vi "BLAS1 Utility(DBL).vi"(0 "x":dbl[](array[numeric]), 1 "y":dbl[](array[numeric]), 2 "xInc":i32, 3 "yInc":i32, 6 "function":T1 items=["ddot/zdotu/zdotc", "daxpy/zaxpy", "dnrm2/dznrm2", "dasum/dzasum", "dcopy/zcopy", "dswap/zswap", "drotm", "drot/zdrot", "idamax/izamax", "idamin/izamin", "dgemv/zgemv", "dsymv/zhemv", "dtrmv/ztrmv", "dsyr/zher", "dsyr2/zher2", "dger/zgeru/zgerc", "dtrsv/ztrsv", "dgemm/zgemm", "dsymm/zsymm/zhemm", "dtrmm/ztrmm", "dsyrk/zsyrk/zherk", "dsyr2k/zsyr2k/zher2k", "dtrsm/ztrsm"]) -> (19 "n":i32)   [LabVIEW 2020, in "NI_AALBLAS.lvlib"]
uses:
  <vilib>/Analysis/NI_AALBLAS.lvlib
  <vilib>/Analysis/BLAS.llb/Fucntion.ctl
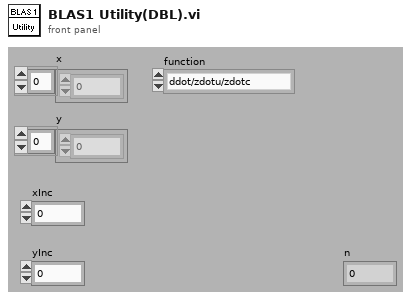
[diagram p1: front panel]
types:
  T1 = typedef "NI_AALBLAS.lvlib/Fucntion.ctl" = u16
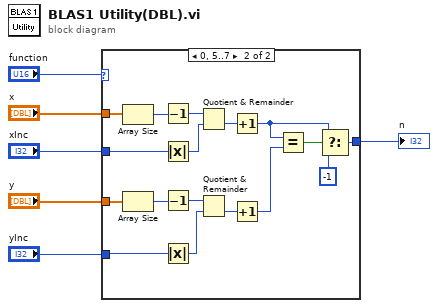
[diagram p0: block diagram]
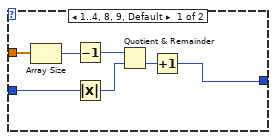
[diagram p2: hidden frame]
diagram:
  n1 = case shown="0, 5..7" "function" {
    tunnel: "x" -> [w13 w30]
    tunnel: "y" -> [_ w29]
    tunnel: [w8 w26] -> w4
    tunnel: "xInc" -> [w10 w24]
    tunnel: "yInc" -> [_ w20]
    frame 1..4, 8, 9, Default {
      n2 = Array Size(array=w13) -> (size(s)=w12:i32)
      n3 = Decrement(x=w12) -> (x-1=w11:i32)
      n4 = Absolute Value(x=w10) -> (abs(x)=w7:i32)
      n5 = Quotient & Remainder(x=w11, y=w7) -> (floor(x/y)=w9:i32)  [unwired: 1 out]
      n6 = Increment(x=w9) -> (x+1=w8:i32)
    }
    frame 0, 5..7 {
      n7 = Array Size(array=w30) -> (size(s)=w25:i32)
      n8 = Array Size(array=w29) -> (size(s)=w21:i32)
      n9 = Decrement(x=w25) -> (x-1=w16:i32)
      n10 = Absolute Value(x=w24) -> (abs(x)=w15:i32)
      n11 = Decrement(x=w21) -> (x-1=w17:i32)
      n12 = Absolute Value(x=w20) -> (abs(x)=w14:i32)
      n13 = Quotient & Remainder(x=w16, y=w15) -> (floor(x/y)=w23:i32)  [unwired: 1 out]
      n14 = Quotient & Remainder(x=w17, y=w14) -> (floor(x/y)=w19:i32)  [unwired: 1 out]
      n15 = Increment(x=w23) -> (x+1=w22:i32)
      n16 = Increment(x=w19) -> (x+1=w18:i32)
      n17 = Equal?(x=w22, y=w18) -> (x = y?=w28:bool)
      n18 = Select(t=w22, s=w28, f=-1) -> (s? t:f=w26:i32)
    }
  }
  "n" <- w4
